vi "Dispatch Sniffer Data.vi"(7 "Data Direction":T1, 8 "error in (no error)":errorcluster, 10 "Data":string, 11 "Stream in":refnum<class "Stream.lvclass">) -> (0 "error out":errorcluster, 3 "Stream out":refnum<class "Stream.lvclass">)   [LabVIEW 2020, in "Stream.lvlib" / "Stream.lvclass"]
uses:
  Stream.lvclass
  Data Direction.ctl
  Stream.lvclass/Stream.ctl
  Endpoint/Endpoint.lvclass
  Stream.lvlib
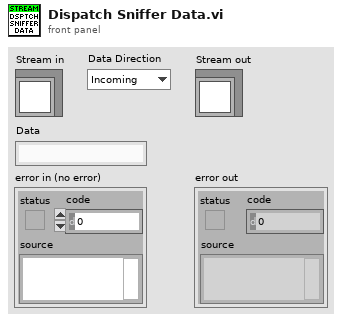
[diagram p1: front panel]
types:
  T1 = typedef "Stream.lvlib/Data Direction.ctl" = enum16{"Incoming", "Outgoing"}
  T2 = typedef "Stream.lvlib/Endpoint.lvclass/State Callback.ctl" = cluster{"Owner":refnum<class>, "VI":refnum<vi>}
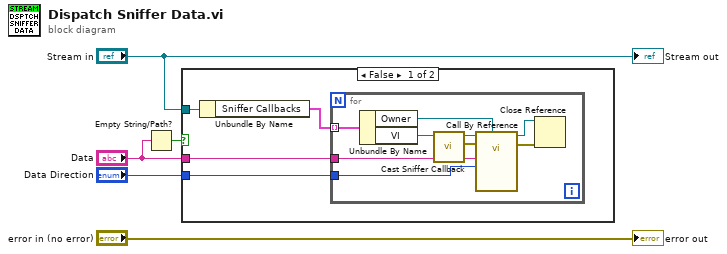
[diagram p0: block diagram]
diagram:
  n1 = Empty String/Path?(string/path="Data") -> (empty?=w1:bool)
  n2 = case shown="False" w1 {
    tunnel: "Stream in" -> [w9 _]
    tunnel: "Data" -> [w7 _]
    tunnel: "Data Direction" -> [w6 _]
    frame False {
      n3 = Unbundle By Name(w9) -> ("Sniffer Callbacks"=w8:T2[])
      n4 = for {
        tunnel: w8 -> [w18] mode=indexing
        tunnel: w7 -> [w13]
        tunnel: w6 -> [w12]
        n5 = Unbundle By Name(w18) -> ("Owner"=w14:refnum<class>, "VI"=w17:refnum<vi>)
        n6 = call "Cast Sniffer Callback.vi"("VI Refnum"=w17) -> ("error out"=w15:errorcluster, "Casted Ref"=w16:refnum<vi>)  [unwired: 9 in]
        n7 = call-by-ref "?"(reference=w16, error in=w15, "Owner"=w14, "Data Direction"=w12, "Data"=w13) -> (reference out=w10:refnum<vi>, error out=w11:errorcluster)  [unwired: 9 in]
        n8 = Close Reference(reference=w10, error in (no error)=w11) -> ()  [unwired: 1 out]
      }
    }
    frame True {
    }
  }
  "error out" <- "error in (no error)"
  "Stream out" <- "Stream in"
